vi "FIR_5decimate_5cycles_for_5761.vi"(7 "reset":bool, 8 "valid in":bool, 10 "Q in":fxp<+/-,16,14>, 11 "I in":fxp<+/-,16,14>) -> (0 "valid out":bool, 2 "Q out":fxp<+/-,16,14>, 3 "I out":fxp<+/-,16,14>, 4 "ready for input":bool)   [LabVIEW 2018]
uses:
  <vilib>/rvi/FXPMathLib/FxpInterpret/XNode/nifxpmath_Interpret.xnode
  <vilib>/fxp/LVFixedPointOverflowPolicyTypeDef.ctl
  <vilib>/fxp/LVFixedPointQuantizationPolicyTypeDef.ctl
  <vilib>/rvi/FXPMathLib/FxpConvert/subVIs/nifxpmath_Convert_SimConfig.ctl
  <vilib>/rvi/FXPMathLib/FxpConvert/simVIs/DllFxpConvertTemp_sub.vi
  <vilib>/rvi/FXPMathLib/FxpConvert/XNode/nifxpmath_Convert.xnode
  <vilib>/rvi/XilinxIP/XIPIN_XNode/niFpgaXIPIN.xnode
  source_from_win7/freia-fast-daq-new/FPGA/Filters_5761/FIR_5decimate_5cycles_for_5761/xsim.dir/FIR_5decimate_5cycles_for_5761_B30259D6F8514136A6E58EBC527CD1D3/xsimk_B30259D6F8514136A6E58EBC527CD1D3.dll
  <vilib>/rvi/IPIntegrationNode/IPINode_Xnode/niFpgaIPINode.xnode
  <vilib>/rvi/IPIntegrationNode/IPINode_Typedef/niFpgaIPINodeSupportedFamilies.ctl
  <vilib>/rvi/IPIntegrationNode/IPINode_Utilities/niFpgaIPINodeSimCore.vi
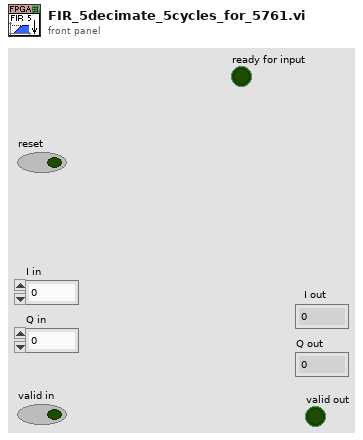
[diagram p1: front panel]
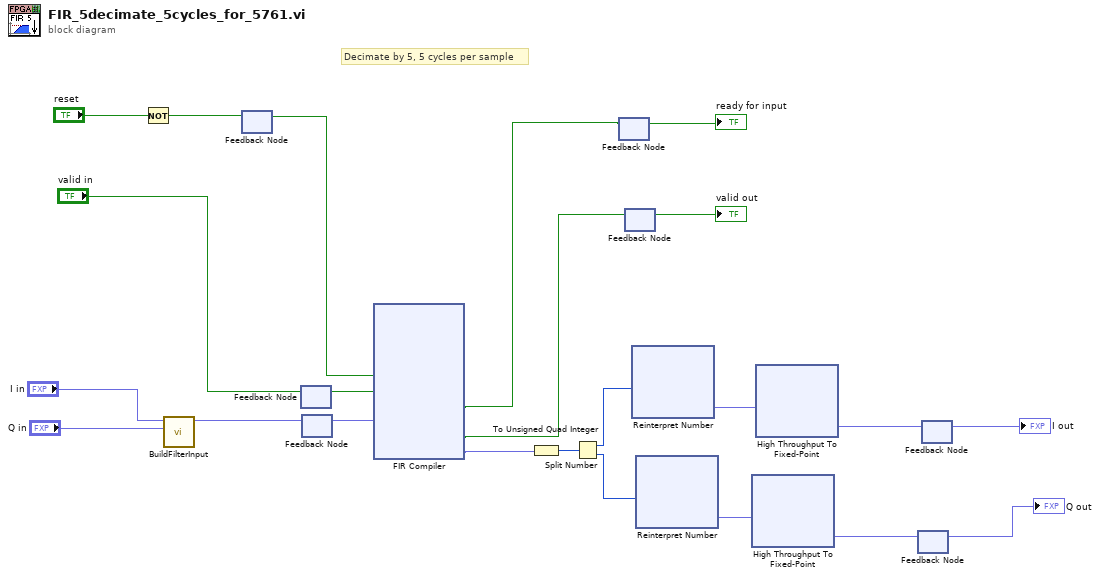
[diagram p0: block diagram]
diagram:
  # "Decimate by 5, 5 cycles per sample"
  n1 = Not(x="reset") -> (.not. x?=w13:bool)
  n2 = call "BuildFilterInput.vi"("Q in"="Q in", "I in"="I in") -> ("Filter input"=w15:fxp<+,32,32>)  [unwired: 9 in]
  n3 = feedback #1() -> (w12:bool)  [unwired: 1 in]
  n4 = feedback-in #1(w13) -> ()
  n5 = feedback #2() -> (w11:bool)  [unwired: 1 in]
  n6 = feedback-in #2("valid in") -> ()
  n7 = feedback-in #3(w15) -> ()
  n8 = feedback #3() -> (w10:fxp<+,32,32>)  [unwired: 1 in]
  n9 = xnode ("FIR Compiler")("aresetn"=w12, "s_axis_data_tvalid"=w11, "s_axis_data_tdata"=w10) -> ("s_axis_data_tready"=w2:bool, "m_axis_data_tvalid"=w4:bool, "m_axis_data_tdata"=w9:fxp<+,64,64>)  [unwired: 1 in]
  n10 = To Unsigned Quad Integer(1:w9) -> (0:w19:u64)
  n11 = Split Number(x=w19) -> (hi(x)=w20:u32, lo(x)=w16:u32)
  n12 = feedback #4() -> (→"ready for input":bool)  [unwired: 1 in]
  n13 = feedback-in #4(w2) -> ()
  n14 = feedback #5() -> (→"valid out":bool)  [unwired: 1 in]
  n15 = feedback-in #5(w4) -> ()
  n16 = xnode "Reinterpret Number"("x"=w20) -> ("y"=w17:fxp<+/-,32,16>)
  n17 = xnode "Reinterpret Number"("x"=w16) -> ("y"=w18:fxp<+/-,32,16>)
  n18 = xnode "High Throughput To Fixed-Point"("x"=w18) -> ("y"=w6:fxp<+/-,16,14>)
  n19 = xnode "High Throughput To Fixed-Point"("x"=w17) -> ("y"=w8:fxp<+/-,16,14>)
  n20 = feedback #6() -> (→"Q out":fxp<+/-,16,14>)  [unwired: 1 in]
  n21 = feedback-in #6(w6) -> ()
  n22 = feedback #7() -> (→"I out":fxp<+/-,16,14>)  [unwired: 1 in]
  n23 = feedback-in #7(w8) -> ()
